vi "Load.vi"(8 "error in (no error)":errorcluster, 10 "Sequence Load Data":T1, 11 "Sequencing in":refnum<class "Sequencing.lvclass">) -> (0 "error out":errorcluster, 3 "Sequencing out":refnum<class "Sequencing.lvclass">)   [LabVIEW 2023, in "VolatusSeq.lvlib" / "Sequencing.lvclass"]
uses:
  Sequencing.lvclass
  Sequence Load Data.ctl
  lv-web-crypto/lv-crypto/Crypto/Hashes/SHA-256/SHA-256.lvclass
  Sequencing.lvclass/Sequencing.ctl
  VolatusErrorUtilities/MultiErrors/MultiErrors.lvclass/MultiErrors.ctl
  VolatusErrorUtilities/MultiErrors/Last Error to Wire.vi
  lv-web-crypto/lv-crypto/Crypto/Crypto.lvlib
  VolatusSeqConfig/Sequence Config/Sequence Config.lvclass
  VolatusErrorUtilities/MultiErrors/MultiErrors.lvclass
  VolatusSeqConfig/Sequence Validation/Sequence Validation.lvclass
  VolatusSeq.lvlib
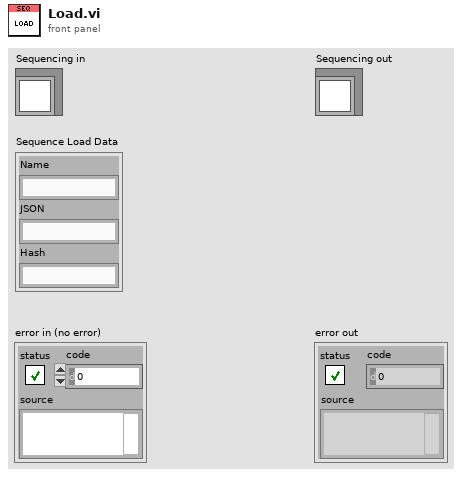
[diagram p1: front panel]
types:
  T1 = typedef "VolatusSeq.lvlib/Sequence Load Data.ctl" = cluster{"Name":string, "JSON":string, "Hash":string}
  T2 = typedef "VolatusSeq.lvlib/Sequence Status.ctl" = cluster{"Name":string, "State":string, "Time":T3, "Running":bool, "Start Time":dbl, "Previous Duration":i64, "Previous Late":bool}
  T3 = typedef "VolatusSeq.lvlib/Sequence Time.ctl" = cluster{"Abort":bool, "Seq Time":dbl, "State Time":dbl, "Wall Time":dbl}
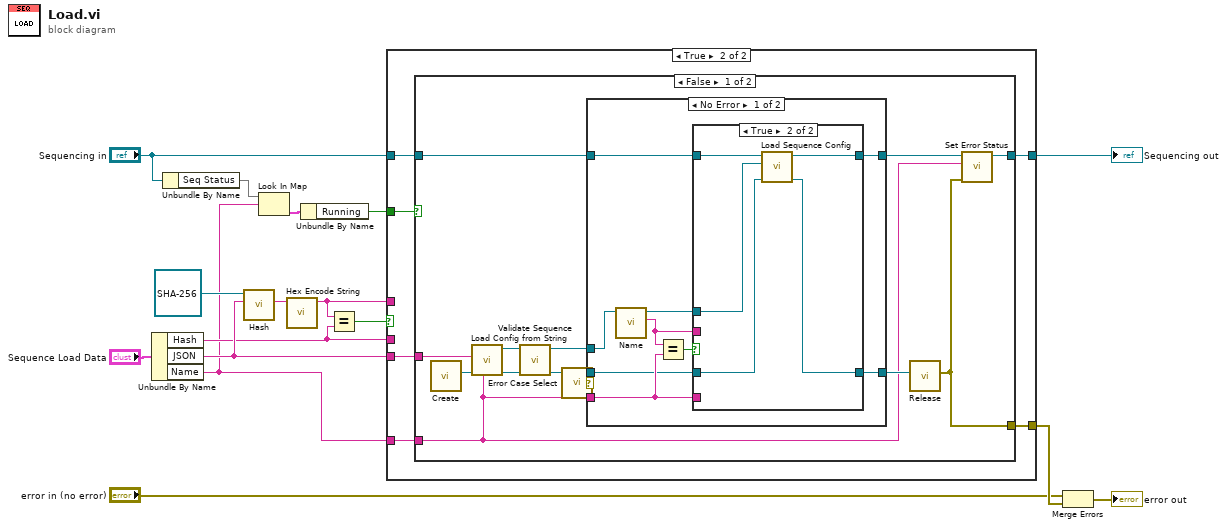
[diagram p0: block diagram]
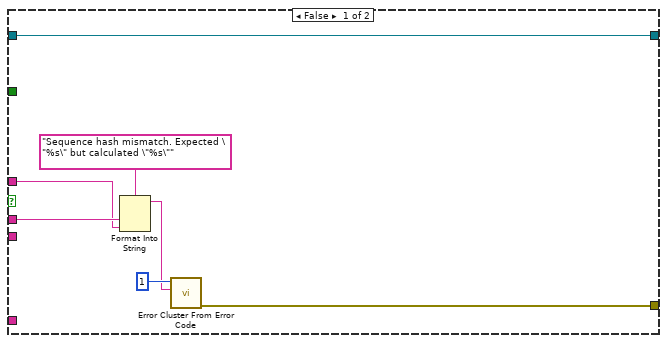
[diagram p2: hidden frame]
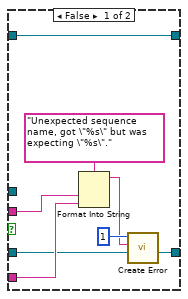
[diagram p3: hidden frame]
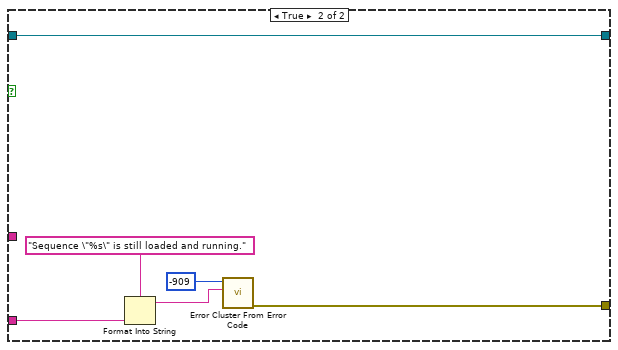
[diagram p5: hidden frame]
diagram:
  n1 = Unbundle By Name("Sequence Load Data") -> ("Hash"=w11:string, "JSON"=w14:string, "Name"=w3:string)
  n2 = Unbundle By Name("Sequencing in") -> ("Seq Status"=w4:map{string, T2})
  n3 = call-dynamic "Hash.vi"("Message"=w14, "SHA-256 in"=refnum<class "SHA-256.lvclass"> refnum ("Crypto.lvlib:SHA-256.lvclass")) -> ("Hash"=w12:string)  [unwired: 7 in, 2 out]
  n4 = Look In Map(map=w4, key=w3) -> (value=w2:T2)  [unwired: 1 in, 1 out]
  n5 = call "Hex Encode String.vi"("String"=w12) -> ("Hex Encoded String"=w10:string)  [unwired: 10 in]
  n6 = Unbundle By Name(w2) -> ("Running"=w1:bool)
  n7 = Equal?(x=w10, y=w11) -> (x = y?=w13:bool)
  n8 = case shown="True" w13 {
    tunnel: w14 -> [_ w29]
    tunnel: w10 -> [w19 _]
    tunnel: w11 -> [w20 _]
    tunnel: [w23 w26] -> w9
    tunnel: "Sequencing in" -> [w23 w27]
    tunnel: [w17 w25] -> w8
    tunnel: w3 -> [_ w28]
    tunnel: w1 -> [_ w24]
    frame False {
      n9 = Format Into String(format string="Sequence hash mismatch. Expected \"%s\" but calculated \"%s\"", w20, w19) -> (resulting string=w18:string)  [unwired: 2 in, 1 out]
      n10 = call <vilib>:"Error Cluster From Error Code.vi"("error message (\"\")"=w18, "error code (0)"=1) -> ("error out"=w17:errorcluster)  [unwired: 7 in]
    }
    frame True {
      n11 = case shown="False" w24 {
        tunnel: w29 -> [w42 _]
        tunnel: w28 -> [w30 w68]
        tunnel: w27 -> [w43 w73]
        tunnel: [w31 w73] -> w26
        tunnel: [w33 w72] -> w25
        frame False {
          n12 = call "Create.vi"() -> ("MultiErrors out"=w41:refnum<class "MultiErrors.lvclass">)  [unwired: 11 in]
          n13 = call "Load Config from String.vi"("Fallback Name"=w30, "error in (no error)"=w41, "JSON"=w42) -> ("error out"=w38:refnum<class "MultiErrors.lvclass">, "Sequence Config"=w37:refnum<class "Sequence Config.lvclass">)  [unwired: 7 in]
          n14 = call "Validate Sequence.vi"("error in (no error)"=w38, "Sequence Config in"=w37) -> ("error out"=w35:refnum<class "MultiErrors.lvclass">, "Sequence Config out"=w36:refnum<class "Sequence Config.lvclass">)  [unwired: 8 in]
          n15 = call "Error Case Select.vi"("MultiErrors in"=w35) -> ("MultiErrors out"=w39:refnum<class "MultiErrors.lvclass">, "error out"=w40:errorcluster)  [unwired: 7 in]
          n16 = case shown="No Error" w40 {
            tunnel: w36 -> [w52 _]
            tunnel: w30 -> [w46 _]
            tunnel: w43 -> [w51 w67]
            tunnel: [w48 w67] -> w32
            tunnel: w39 -> [w45 w66]
            tunnel: [w44 w66] -> w34
            frame No Error {
              n17 = call "Name.vi"("Sequence Config in"=w52) -> ("Name"=w47:string, "Sequence Config out"=w49:refnum<class "Sequence Config.lvclass">)  [unwired: 8 in, 1 out]
              n18 = Equal?(x=w47, y=w46) -> (x = y?=w50:bool)
              n19 = case shown="True" w50 {
                tunnel: w51 -> [w60 w65]
                tunnel: w49 -> [_ w62]
                tunnel: [w60 w64] -> w48
                tunnel: w47 -> [w59 _]
                tunnel: w46 -> [w58 _]
                tunnel: [w53 w61] -> w44
                tunnel: w45 -> [w54 w63]
                frame False {
                  n20 = Format Into String(format string="Unexpected sequence name, got \"%s\" but was expecting \"%s\".", w59, w58) -> (resulting string=w55:string)  [unwired: 2 in, 1 out]
                  n21 = call "Create Error.vi"("MultiErrors in"=w54, "Message"=w55, "Code"=1 ("error code (0)")) -> ("MultiErrors out"=w53:refnum<class "MultiErrors.lvclass">)  [unwired: 8 in]
                }
                frame True {
                  n22 = call "Load Sequence Config.vi"("error in (no error)"=w63, "Sequence Config"=w62, "Sequencing in"=w65) -> ("error out"=w61:refnum<class "MultiErrors.lvclass">, "Sequencing out"=w64:refnum<class "Sequencing.lvclass">)  [unwired: 7 in]
                }
              }
            }
            frame Error {
            }
          }
          n23 = call "Release.vi"("MultiErrors in"=w34) -> ("error out"=w33:errorcluster)  [unwired: 10 in]
          n24 = call "Set Error Status.vi"("error in (no error)"=w33, "Sequence"=w30, "Sequencing in"=w32) -> ("Sequencing out"=w31:refnum<class "Sequencing.lvclass">)  [unwired: 7 in, 1 out]
        }
        frame True {
          n25 = Format Into String(format string="Sequence \"%s\" is still loaded and running.", w68) -> (resulting string=w69:string)  [unwired: 2 in, 1 out]
          n26 = call <vilib>:"Error Cluster From Error Code.vi"("error message (\"\")"=w69, "error code (0)"=-909) -> ("error out"=w72:errorcluster)  [unwired: 7 in]
        }
      }
    }
  }
  "Sequencing out" <- w9
  n27 = Merge Errors("error in (no error)", w8) -> (→"error out":errorcluster)
